vi "Inst.RP100.setStrain.vi"(8 "error in (no error)":errorcluster, 10 "data in":variant, 11 "Inst.RP100 in":refnum<class "Inst.RP100.lvclass">) -> (0 "error out":errorcluster, 3 "Inst.RP100 out":refnum<class "Inst.RP100.lvclass">)   [LabVIEW 2019, in "Inst.RP100.lvlib" / "Inst.RP100.lvclass"]
uses:
  Inst.RP100.lvclass
  Typedefs/Channel--Num.ctl
  Typedefs/State--Enum.ctl
  <userlib>/LevyLab/Instrument Framework/Instrument Types/Strain/Typedefs/setStrain--cluster.ctl
  Inst.RP100.lvclass/Inst.RP100.ctl
  0e620bb2-1128-41c0-862e-a3f78ee0742e.vi
  0e620bb2-1128-41c0-862e-a3f78ee0742e.vi/4ef606d9-0162-4704-994d-678fb990cc6a.vi
  0e620bb2-1128-41c0-862e-a3f78ee0742e.vi/9ced8730-bfe8-4cc4-bfd9-7aa359bffdc7.vi
  <vilib>/Utility/Data Type/Get Type Information.vi
  <vilib>/JDP Science/JSONtext/JSON text to Variant.vi
  <vilib>/JDP Science/JSONtext/LVClass Serializer/JSONtext LVClass Serializer.lvclass
  RP100/RP100.lvlib
  <userlib>/LevyLab/Instrument Framework/Instrument Types/Strain/Instrument.Strain.lvclass
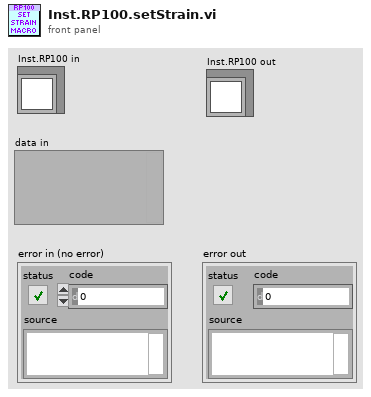
[diagram p1: front panel]
types:
  T1 = typedef "Instrument.Strain.lvclass/setStrain--cluster.ctl" = cluster{"strain":dbl, "slew":dbl, "channel":i32}
  T2 = typedef "Inst.RP100.lvlib/Inst.RP100.lvclass/Channel--Num.ctl" = i32
  T3 = typedef "Inst.RP100.lvlib/Inst.RP100.lvclass/State--Enum.ctl" = enum16{"Shorted", "Enabled"}
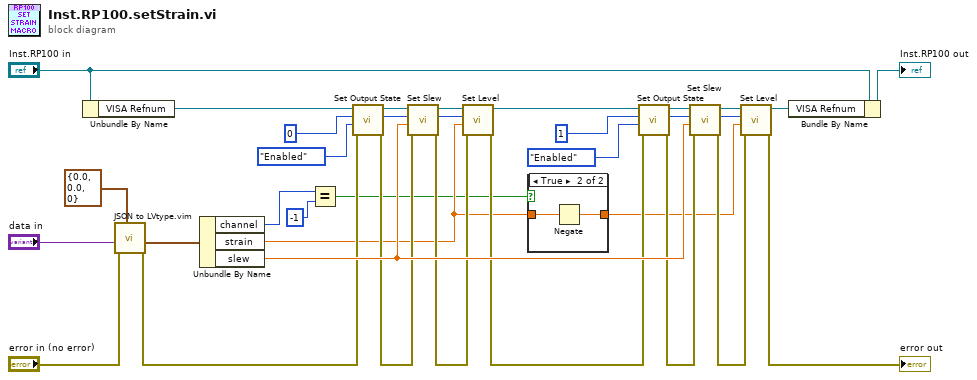
[diagram p0: block diagram]
diagram:
  n1 = Unbundle By Name("Inst.RP100 in") -> ("VISA Refnum"=w14:refnum<visa-resource-name>)
  n2 = call "JSON to LVtype.vim"("type"=T1 {"strain"=0.0, "slew"=0.0, "channel"=0} ("setStrain"), "error in (no error)"="error in (no error)", "JSON Data in"="data in") -> ("error out"=w6:errorcluster, "Data out"=w9:T1)  [unwired: 7 in]
  n3 = Unbundle By Name(w9) -> ("channel"=w1:i32, "strain"=w4:dbl, "slew"=w30:dbl)
  n4 = Equal?(x=w1, y=-1) -> (x = y?=w2:bool)
  n5 = call "Set Output State.vi"("error in (no error)"=w6, "Output State"=State--Enum."Enabled", "Output Channel"=T2 0, "VISA resource name"=w14) -> ("error out"=w18:errorcluster, "Output Channel"=w25:T2, "VISA Refnum out"=w24:refnum<visa-resource-name>)  [unwired: 5 in]
  n6 = call "Set Slew.vi"("error in (no error)"=w18, "Slew (V/s)"=w30, "Output Channel"=w25, "VISA resource name"=w24) -> ("error out"=w19:errorcluster, "Output Channel"=w26:T2, "VISA Refnum out"=w27:refnum<visa-resource-name>)  [unwired: 5 in]
  n7 = call "Set Level.vi"("error in (no error)"=w19, "Level (V)"=w4, "Output Channel"=w26, "VISA resource name"=w27) -> ("error out"=w20:errorcluster, "VISA Refnum out"=w28:refnum<visa-resource-name>)  [unwired: 5 in, 1 out]
  n8 = case shown="True" w2 {
    tunnel: w4 -> [w35 w37]
    tunnel: [w35 w36] -> w3
    frame False {
    }
    frame True {
      n9 = Negate(x=w37) -> (-x=w36:dbl)
    }
  }
  n10 = call "Set Output State.vi"("error in (no error)"=w20, "Output State"=State--Enum."Enabled", "Output Channel"=T2 1, "VISA resource name"=w28) -> ("error out"=w21:errorcluster, "Output Channel"=w29:T2, "VISA Refnum out"=w33:refnum<visa-resource-name>)  [unwired: 5 in]
  n11 = call "Set Slew.vi"("error in (no error)"=w21, "Slew (V/s)"=w30, "Output Channel"=w29, "VISA resource name"=w33) -> ("error out"=w22:errorcluster, "Output Channel"=w31:T2, "VISA Refnum out"=w32:refnum<visa-resource-name>)  [unwired: 5 in]
  n12 = call "Set Level.vi"("error in (no error)"=w22, "Level (V)"=w3, "Output Channel"=w31, "VISA resource name"=w32) -> ("error out"=→"error out":errorcluster, "VISA Refnum out"=w13:refnum<visa-resource-name>)  [unwired: 5 in, 1 out]
  n13 = Bundle By Name(cluster="Inst.RP100 in", "VISA Refnum"=w13) -> (→"Inst.RP100 out":refnum<class "Inst.RP100.lvclass">)
